vi "RSNRPZ Set Correction Frequency.vi"(8 "error in (no error)":errorcluster, 9 "Frequency ( 50.0e6 Hz)":dbl=50000000.0 format="%.2p", 10 "Channel (1)":i32=1, 11 "VISA session":refnum<visa-resource-name> caption="VISA resource name") -> (0 "error out":errorcluster, 3 "dup VISA session":refnum<visa-resource-name> caption="VISA resource name")   [LabVIEW 2019]
doc: "This VI informs the R&S NRP about the frequency of the power to be measured since this frequency is not automatically determined. The frequency is used to determine a frequency-dependent correction factor for the measurement results.\n\nRemote-control command(s):\nSENS:FREQ"
uses:
  rsnrpz_32.dll
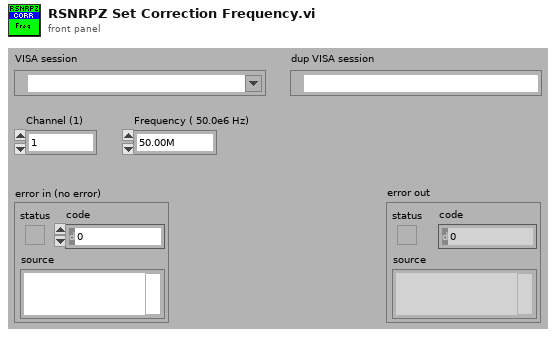
[diagram p1: front panel]
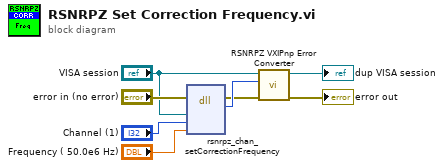
[diagram p0: block diagram]
diagram:
  n1 = dll-call lib="C:/Users/LABadmin/Documents/Jarvis/user_lib/rsnrpz/rsnrpz_32.dll" fn="rsnrpz_chan_setCorrectionFrequency"(error in="error in (no error)", "VISA Session"="VISA session", "Channel"="Channel (1)", "Frequency"="Frequency ( 50.0e6 Hz)") -> (error out=w5:errorcluster, "Status"=w8:i32)  [unwired: 5 in, 1 out]
  n2 = call <instrlib>:"RSNRPZ VXIPnp Error Converter.vi"("error in"=w5, "VXIPnp error code"=w8, "VISA session"="VISA session") -> ("error out"=→"error out":errorcluster, "dup VISA session"=→"dup VISA session":refnum<visa-resource-name>)  [unwired: 7 in]
